vi "demo.vi"() -> ()   [LabVIEW 2013, in "Tag Data by Variant.lvlib"]
uses:
  Tag Data by Variant.lvlib
  Custom def/Tag DBL.ctl
  Custom def/Tag Boolean.ctl
  Init/Init(DBL).vi
  Init/Init(Boolean).vi
  Read All/ReadAll(DBL).vi
  Add/Add(Boolean).vi
  Read/Read(Boolean).vi
  Add/Add(DBL).vi
panel:
  out "TagDataArray":T1[](array[typedef])
  in  "停止":bool
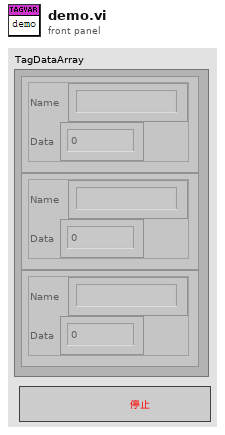
[diagram p1: front panel]
types:
  T1 = typedef "Tag Data by Variant.lvlib/Tag DBL.ctl" = cluster{"Name":string, "Data":dbl}
  T2 = typedef "Tag Data by Variant.lvlib/Tag Boolean.ctl" = cluster{"Name":string, "Data":bool}
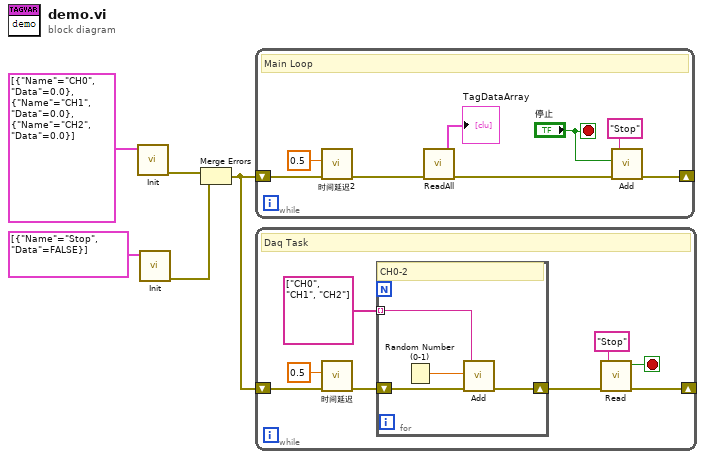
[diagram p0: block diagram]
diagram:
  n1 = call-poly "Init.vi"("TagList"=T1[] [{"Name"="CH0", "Data"=0.0}, {"Name"="CH1", "Data"=0.0}, {"Name"="CH2", "Data"=0.0}]) -> ("错误输出"=w3:errorcluster)  [unwired: 10 in]
  n2 = call-poly "Init.vi"("TagList"=T2[] [{"Name"="Stop", "Data"=FALSE}]) -> ("错误输出"=w2:errorcluster)  [unwired: 10 in]
  n3 = Merge Errors(w3, w2) -> (w1:errorcluster)
  n4 = while {
    shift-right: [w6] -> _
    shift-left: w1 -> [w13]
    stop <- "停止" stop-if-true
    # "Main Loop"
    n5 = call "时间延迟2"("error in (no error)"=w13, "Delay Time (s)"=0.5) -> ("error out"=w11:errorcluster)  [unwired: 9 in]
    n6 = call-poly "ReadAll.vi"("错误输入"=w11) -> ("错误输出"=w9:errorcluster, "TagDataArray"=→"TagDataArray":T1[])  [unwired: 9 in]
    n7 = call-poly "Add.vi"("错误输入"=w9, "Value"="停止", "TagName"="Stop") -> ("错误输出"=w6:errorcluster)  [unwired: 8 in]
  }
  n8 = while {
    shift-right: [w16] -> _
    shift-left: w1 -> [w21]
    stop <- w17 stop-if-true
    # "Daq Task"
    n9 = call "时间延迟"("error in (no error)"=w21, "Delay Time (s)"=0.5) -> ("error out"=w19:errorcluster)  [unwired: 9 in]
    n10 = for {
      tunnel: string[] ["CH0", "CH1", "CH2"] -> [w23] mode=indexing
      shift-right: [w22] -> w14
      shift-left: w19 -> [w25]
      # "CH0-2"
      n11 = Random Number (0-1)() -> (number: 0 to 1=w24:dbl)
      n12 = call-poly "Add.vi"("错误输入"=w25, "Value"=w24, "TagName"=w23) -> ("错误输出"=w22:errorcluster)  [unwired: 8 in]
    }
    n13 = call-poly "Read.vi"("错误输入"=w14, "TagName"="Stop") -> ("错误输出"=w16:errorcluster, "Data"=w17:bool)  [unwired: 8 in]
  }
